vi "MatrixSwitchSingle.vi"(7 "Switch action":u16(ring) items=["Open", "Close"], 8 "error in (no error)":errorcluster, 9 "Matrix Y":i32=1 min=1 max=12 step=1, 10 "Matrix X":i32=1 min=1 max=12 step=1, 11 "Pickering in":refnum<class "PickeringPrague.lvclass">) -> (0 "error out":errorcluster, 2 "command string":string, 3 "Pickering out":refnum<class "PickeringPrague.lvclass">)   [LabVIEW 2018, in "PickeringPrague.lvclass"]
uses:
  PickeringPrague.lvclass
  C:/Users/itk/Documents/itk-strip-sensor-qc/InstrControl/InstrControl.lvclass
  PickeringMatrix_CommandsGlobal.vi
  InstrControl.lvclass
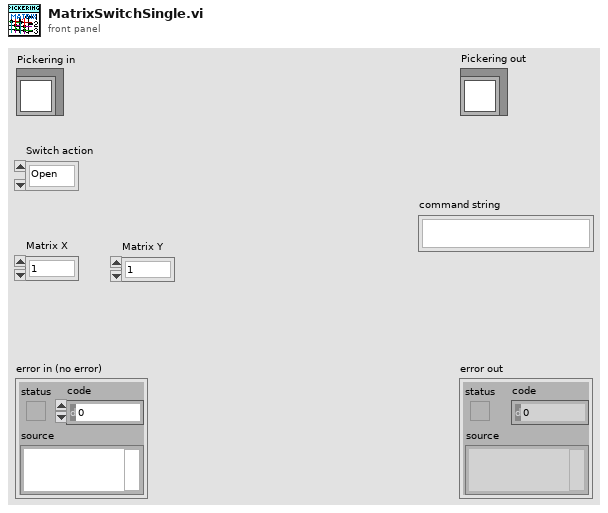
[diagram p1: front panel]
types:
  T1 = cluster{"Matrix address":string, "Instrument name":string, "Instrument type":u16, "Command \"Matrix Reset\"":string, "Command \"Connect Matrix Channels\"":string, "Command \"Disconnect Matrix Channels\"":string}
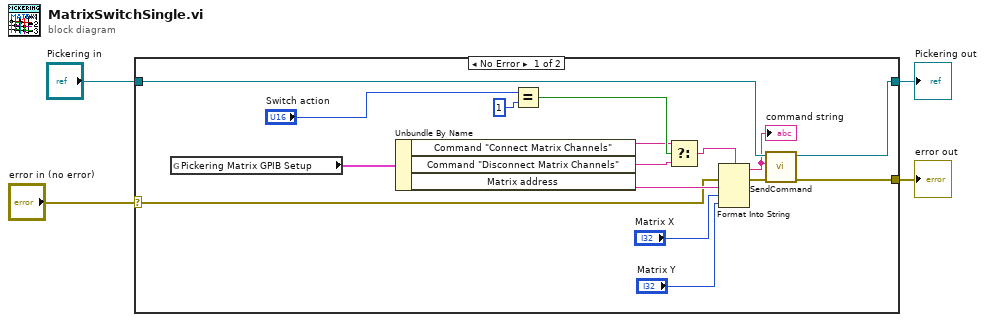
[diagram p0: block diagram]
diagram:
  n1 = case shown="No Error" "error in (no error)" {
    selector: "error in (no error)" -> [w13 w22]
    tunnel: "Pickering in" -> [w9 w21]
    tunnel: [w11 w22] -> w2
    tunnel: [w10 w21] -> w1
    frame No Error {
      n2 = global read "PickeringMatrix_CommandsGlobal.vi" "Pickering Matrix GPIB Setup"() -> (w18:T1)
      n3 = Unbundle By Name(w18) -> ("Command \"Connect Matrix Channels\""=w16:string, "Command \"Disconnect Matrix Channels\""=w15:string, "Matrix address"=w14:string)
      n4 = Equal?(x="Switch action", y=1) -> (x = y?=w17:bool)
      n5 = Select(t=w16, s=w17, f=w15) -> (s? t:f=w6:string)
      n6 = Format Into String(format string=w6, error in=w13, w14, "Matrix X", "Matrix Y") -> (resulting string=w5:string, error out=w12:errorcluster)  [unwired: 1 in]
      "command string" <- w5
      n7 = call "SendCommand.vi"("error in (no error)"=w12, "Command string"=w5, "InstControl in"=w9) -> ("error out"=w11:errorcluster, "InstControl out"=w10:refnum<class "PickeringPrague.lvclass">)  [unwired: 7 in]
    }
    frame Error {
    }
  }
  "error out" <- w2
  "Pickering out" <- w1
